vi "Hopping step(linear-XZ).vi"() -> ()   [LabVIEW 2014]
uses:
  <vilib>/Platform/TimedLoop/XDataNode/timing_clust.ctl
  <vilib>/Platform/TimedLoop/XDataNode/nitl_modes.ctl
  <vilib>/Platform/TimedLoop/XDataNode/wakeup.ctl
  <vilib>/rvi/Emulation/niFpgaGetClockAttributes.vi
  <vilib>/rvi/Emulation/niFpgaSctlEmulationGetInTimedLoop.vi
  <vilib>/rvi/Emulation/niFpgaEmulationReportErrorSimple.vi
  <vilib>/rvi/eio/common/nirviEmuTemplateMethod_errors.vi
  <vilib>/rvi/Emulation/niFpgaCriticalErrorInLSC.vi
  <vilib>/rvi/interface/RandomDataEmulation/niFpgaRandomDataHandleErrors.vi
  <vilib>/rvi/Emulation/niFpgaProcessEmulError.vi
  <vilib>/eio/EIONode/EIONode.xnode
  <vilib>/Platform/TimedLoop/XDataNode/XDataNode.xnode
  <vilib>/rvi/DataTransferAndStorage/Container/XNode/niFpgaContainer.xnode
  <vilib>/rvi/interface/RandomDataEmulation/nirviRandomDataFpgaReadWriteTemplate.vi
  <vilib>/Platform/TimedLoop/XDataNode/XDNodeRunTimeDep.lvlib
panel:
  out "Waveform Chart":i32(graph)
  out "ZRealPos":i16
  in  "stop":bool
  out "Z":i32(graph)
  in  "ZOffset":i16
  in  "XNum":i16
  in  "XOffset":i16
  in  "XStepIndex":i16
  in  "WhetherDoubleRow?":bool=TRUE
  in  "RelativeWithdraw":i16
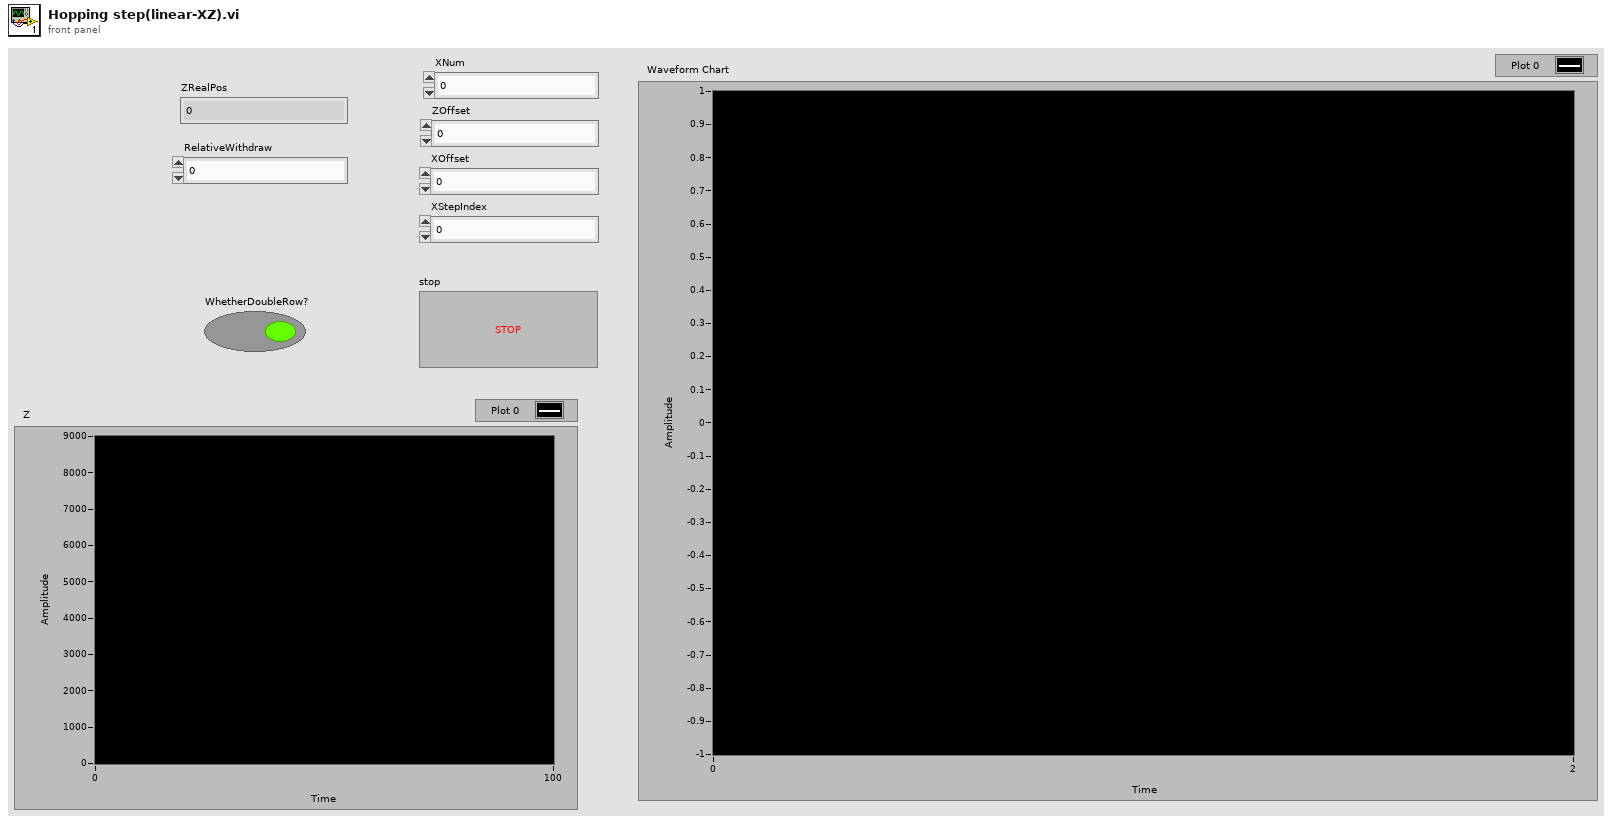
[diagram p1: front panel]
types:
  T1 = typedef "XDNodeRunTimeDep.lvlib/timing_clust.ctl" = cluster{"Expected End [f-1]":u64, "Actual End [f-1]":u64, "Finished Late? [f-1]":bool, "Expected End [i-1]":u64, "Actual End [i-1]":u64, "Finished Late? [i-1]":bool, "Expected Start [i]":u64, "Actual Start [i]":u64, "Expected Start [f]":u64, "Actual Start [f]":u64, "Source Name":string, "Structure Name":string, "Period":i64, "Deadline":i64, "Offset":i64, "Start":i64, "Priority":i32, "Timeout":i32, "Mode":T2, "Wakeup Reason":T3, "Error":errorcluster, "Source Type":string, "Secondary Source Type":string, "Global End Time":u64, "Global Start Time":u64, "Frame Duration":u64, "Iteration Duration":u64, "Assigned CPU":i32, "I/O Scan Engine Mode":u32}
  T2 = typedef "XDNodeRunTimeDep.lvlib/nitl_modes.ctl" = enum32{"No Change", "Process missed periods, maintain original phase", "Discard missed periods, maintain original phase", "Process missed periods, ignore original phase", "Discard missed periods, ignore original phase"}
  T3 = typedef "XDNodeRunTimeDep.lvlib/wakeup.ctl" = enum32{"Normal", "Aborted", "Asynchronous wakeup", "Timing source error", "Timed loop error", "Timeout"}
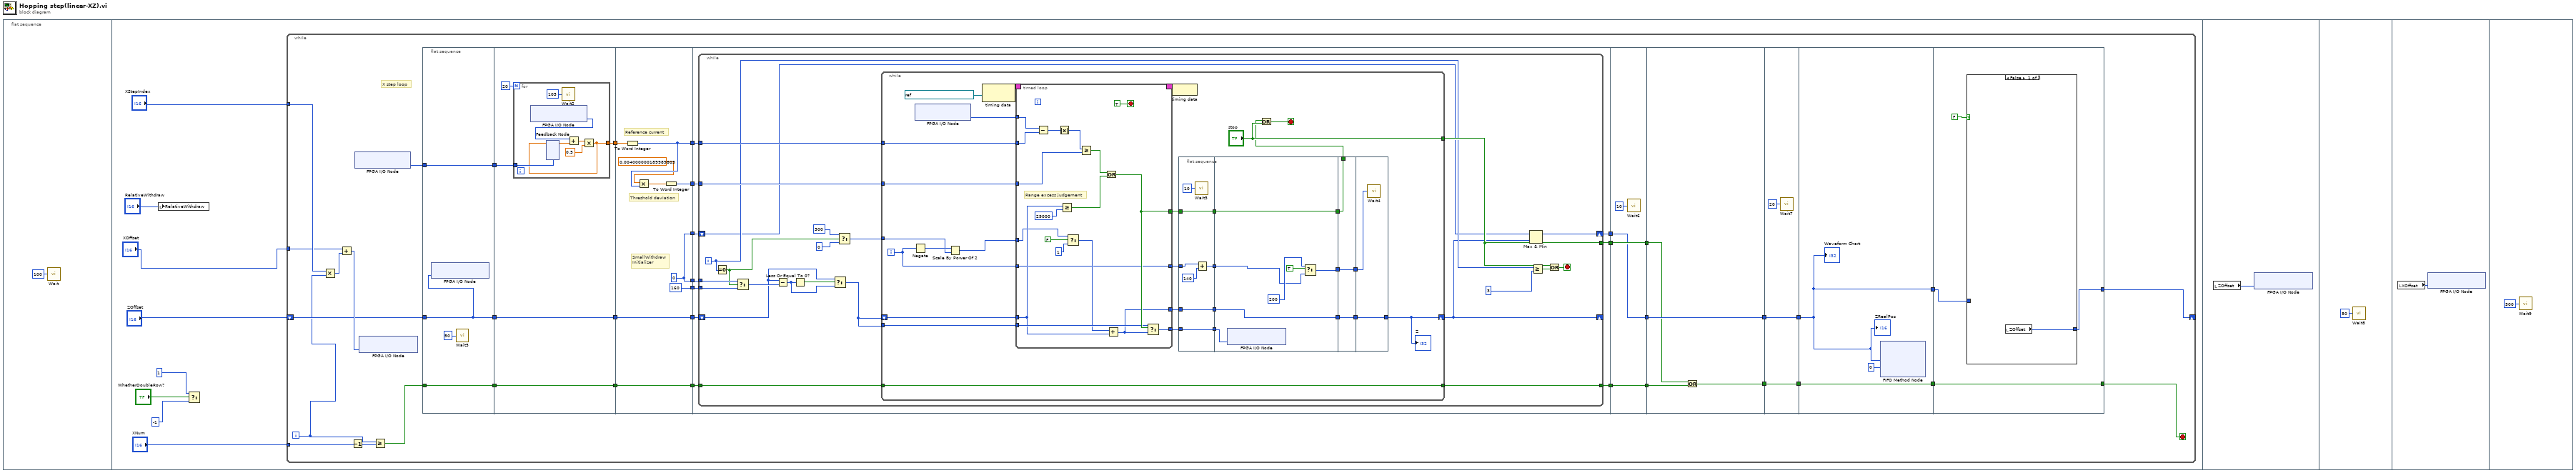
[diagram p0: block diagram]
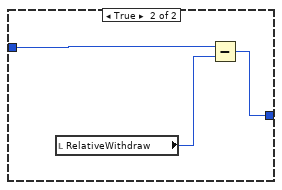
[diagram p2: hidden frame]
diagram:
  n1 = flat-sequence {
    frame #0 {
      n2 = call "Wait"("Count(mSec)"=u32 100 ("Count(uSec)")) -> ()  [unwired: 1 out]
    }
    frame #1 {
      n3 = local write "RelativeWithdraw"("RelativeWithdraw") -> ()
      n4 = Select(t=i16 1, s="WhetherDoubleRow?", f=i16 -1) -> ()  [unwired: 1 out]
      n5 = while {
        tunnel: "XNum" -> [w22]
        tunnel: "XStepIndex" -> [w23]
        shift-right: [w10] -> _
        shift-left: "ZOffset" -> [w24]
        tunnel: "XOffset" -> [w13]
        i -> [w14]
        stop <- w33 stop-if-true
        # "X step loop"
        n6 = Multiply(x=w23, y=w14) -> (x*y=w28:i32)
        n7 = Add(x=w13, y=w28) -> (x+y=w29:i32)
        n8 = Decrement(x=w22) -> (x-1=w21:i16)
        n9 = xnode "FPGA I/O Node"() -> ("Connector0/AI1"=w40:i16)  [unwired: 1 in, 1 out]
        n10 = xnode "FPGA I/O Node"("Connector0/AO2"=w29) -> ()  [unwired: 1 in, 1 out]
        n11 = Greater Or Equal?(x=w14, y=w21) -> (x >= y?=w20:bool)
        n12 = flat-sequence {
          tunnel: [w49] -> w45
          tunnel: w40 -> [w49]
          tunnel: [w48] -> w30
          tunnel: w24 -> [w48]
          tunnel: w20 -> [w47]
          tunnel: [w47] -> w19
          tunnel: w45 -> [w55]
          tunnel: [w53] -> w44
          tunnel: [w52] -> w31
          tunnel: w30 -> [w52]
          tunnel: w19 -> [w51]
          tunnel: [w51] -> w18
          tunnel: [w65] -> w46
          tunnel: w44 -> [w71]
          tunnel: [w70] -> w43
          tunnel: [w67] -> w42
          tunnel: [i16 160] -> w32
          tunnel: w31 -> [w65]
          tunnel: [w64] -> w27
          tunnel: [w64] -> w26
          tunnel: w18 -> [w63]
          tunnel: [w63] -> w17
          tunnel: w42 -> [w79]
          tunnel: w43 -> [w80]
          tunnel: w46 -> [w81]
          tunnel: [w78] -> w36
          tunnel: w32 -> [w77]
          tunnel: w27 -> [w76]
          tunnel: w26 -> [w75]
          tunnel: [w74] -> w25
          tunnel: w17 -> [w73]
          tunnel: [w72] -> w15
          tunnel: [w180] -> w41
          tunnel: [w181] -> w37
          tunnel: w36 -> [w181]
          tunnel: w25 -> [w180]
          tunnel: [w179] -> w16
          tunnel: w15 -> [w179]
          tunnel: w41 -> [w186]
          tunnel: [w186] -> w39
          tunnel: w37 -> [w185]
          tunnel: [w184] -> w34
          tunnel: w16 -> [w183]
          tunnel: w39 -> [w188]
          tunnel: [w188] -> w38
          tunnel: [w187] -> w35
          tunnel: w34 -> [w187]
          tunnel: w38 -> [w190]
          tunnel: w35 -> [w191]
          tunnel: [w191] -> w12
          tunnel: [w190] -> w11
          tunnel: [w194] -> w10
          tunnel: [w196] -> w33
          tunnel: w12 -> [w196]
          tunnel: w11 -> [w193]
          frame #0 {
            n13 = xnode "FPGA I/O Node"("Connector0/AO0"=w48) -> ()  [unwired: 1 in, 1 out]
            n14 = call "Wait5"("Count(uSec)"=u32 50) -> ()  [unwired: 1 out]
          }
          frame #1 {
            n15 = for {
              N: 20 -> [_]
              tunnel: w55 -> [w61]
              tunnel: [w56] -> w53
              n16 = xnode "FPGA I/O Node"() -> ("Connector0/AI1"=w59:i16)  [unwired: 1 in, 1 out]
              n17 = feedback #1(w61) -> (w60:sgl)
              n18 = call "Wait2"("Count(uSec)"=u32 105) -> ()  [unwired: 1 out]
              n19 = Add(x=w59, y=w60) -> (x+y=w58:sgl)
              n20 = Multiply(x=w58, y=sgl 0.5) -> (x*y=w56:sgl)
              n21 = feedback-in #1(w56) -> ()
            }
          }
          frame #2 {
            w64 = i16 0
            # "SmallWithdraw\nInitializer"
            # "Threshold deviation"
            # "Reference current"
            n22 = To Word Integer(number=w71) -> (16bit integer=w70:i16)
            n23 = Multiply(x=sgl 0.004, y=w70) -> (x*y=w68:sgl)
            n24 = To Word Integer(number=w68) -> (16bit integer=w67:i16)
          }
          frame #3 {
            n25 = while {
              tunnel: w80 -> [w104]
              tunnel: w79 -> [w103]
              tunnel: [w100] -> w78
              tunnel: w77 -> [w98]
              shift-right: [w90] -> _
              shift-left: w81 -> [w95]
              tunnel: w76 -> [w92]
              shift-right: [w89] -> w74
              shift-left: w75 -> [w91]
              tunnel: w73 -> [w85]
              tunnel: [w84] -> w72
              i -> [w99]
              stop <- w102 stop-if-true
              n26 = Equal To 0?(x=w99) -> (x = 0?=w82:bool)
              n27 = Select(t=w92, s=w82, f=w98) -> (s? t:f=w97:i16)
              n28 = Subtract(x=w95, y=w97) -> (x-y=w94:i32)
              n29 = Less Or Equal To 0?(x=w94) -> (x <= 0?=w96:bool)
              n30 = Select(t=w95, s=w96, f=w94) -> (s? t:f=w93:i32)
              n31 = Select(t=i16 300, s=w82, f=i16 0) -> (s? t:f=w86:i16)
              n32 = while {
                tunnel: w104 -> [w127]
                tunnel: w103 -> [w129]
                tunnel: ["stop"] -> w100
                shift-right: [w118] -> w90
                shift-left: w93 -> [w124]
                tunnel: w93 -> [w121]
                tunnel: w86 -> [w108]
                tunnel: w85 -> [w105]
                tunnel: [w105] -> w84
                i -> [w106]
                stop <- w131 stop-if-true
                n33 = Negate(x=w106) -> (-x=w109:i32)
                n34 = xnode "FPGA I/O Node"() -> ("Connector0/AI1"=w128:i16)  [unwired: 1 in, 1 out]
                n35 = Scale By Power Of 2(n=w109, x=w108) -> (x*2^n=w107:i16)
                n36 = node-c288(refnum<k21> "40 MHz Onboard Clock" ("Source Name")) -> (w134:T1)
                n37 = timed-loop {
                  timing: w134 -> [_]
                  timing-out: [_] -> w133
                  tunnel: w127 -> [w170]
                  tunnel: w129 -> [w156]
                  tunnel: w128 -> [w171]
                  tunnel: [w166] -> w125
                  tunnel: [w165] -> w123
                  tunnel: w124 -> [w162]
                  tunnel: w121 -> [w164]
                  tunnel: [w161] -> w120
                  tunnel: w107 -> [w157]
                  tunnel: [w158] -> w110
                  tunnel: w106 -> [w158]
                  stop <- TRUE stop-if-true
                  # "Range excess judgement"
                  n38 = Subtract(x=w171, y=w170) -> (x-y=w155:i16)
                  n39 = Absolute Value(x=w155) -> (abs(x)=w169:i16)
                  n40 = Greater Or Equal?(x=w162, y=i16 29000) -> (x >= y?=w167:bool)
                  n41 = Select(t=w157, s=FALSE, f=1) -> (s? t:f=w159:i32)
                  n42 = Greater Or Equal?(x=w169, y=w156) -> (x >= y?=w168:bool)
                  n43 = Or(x=w168, y=w167) -> (x .or. y?=w165:bool)
                  n44 = Add(x=w159, y=w162) -> (x+y=w161:i32)
                  n45 = Select(t=w164, s=w165, f=w161) -> (s? t:f=w166:i32)
                }
                n46 = node-c288(w133) -> ()
                n47 = flat-sequence {
                  tunnel: [w140] -> w126
                  tunnel: w125 -> [w140]
                  tunnel: w123 -> [w139]
                  tunnel: [w139] -> w122
                  tunnel: w120 -> [w138]
                  tunnel: [w138] -> w119
                  tunnel: [w136] -> w111
                  tunnel: w110 -> [w137]
                  tunnel: w126 -> [w146]
                  tunnel: [w148] -> w117
                  tunnel: w122 -> [w147]
                  tunnel: w119 -> [w148]
                  tunnel: [w147] -> w115
                  tunnel: [w144] -> w112
                  tunnel: w111 -> [w143]
                  tunnel: w117 -> [w151]
                  tunnel: [w151] -> w116
                  tunnel: w115 -> [w150]
                  tunnel: [w150] -> w114
                  tunnel: [w149] -> w113
                  tunnel: w112 -> [w149]
                  tunnel: w116 -> [w153]
                  tunnel: [w153] -> w118
                  tunnel: w113 -> [w152]
                  frame #0 {
                    n48 = call "Wait3"("Count(uSec)"=u32 10) -> ()  [unwired: 1 out]
                    n49 = Add(x=w137, y=140) -> (x+y=w136:i32)
                  }
                  frame #1 {
                    n50 = xnode "FPGA I/O Node"("Connector0/AO0"=w146) -> ()  [unwired: 1 in, 1 out]
                    n51 = Select(t=i16 200, s=TRUE, f=w143) -> (s? t:f=w144:i32)
                  }
                  frame #2 {
                  }
                  frame #3 {
                    n52 = call "Wait4"("Count(uSec)"=w152) -> ()  [unwired: 1 out]
                  }
                }
                n53 = Or(x=w114, y="stop") -> (x .or. y?=w131:bool)
                "Z" <- w118
              }
              n54 = Max & Min(x=w91, y=w90) -> (max(x,y)=w89:i32)  [unwired: 1 out]
              n55 = Greater Or Equal?(x=w99, y=3) -> (x >= y?=w101:bool)
              n56 = Or(x=w100, y=w101) -> (x .or. y?=w102:bool)
            }
          }
          frame #4 {
            n57 = call "Wait6"("Count(uSec)"=u32 10) -> ()  [unwired: 1 out]
          }
          frame #5 {
            n58 = Or(x=w185, y=w183) -> (x .or. y?=w184:bool)
          }
          frame #6 {
            n59 = call "Wait7"("Count(uSec)"=u32 20) -> ()  [unwired: 1 out]
          }
          frame #7 {
            n60 = xnode ("FIFO Method Node")("Element"=w190, "Timeout"=0) -> ()  [unwired: 1 in, 2 out]
            "Waveform Chart" <- w190
            "ZRealPos" <- w190
          }
          frame #8 {
            n61 = case shown="False" FALSE {
              tunnel: w193 -> [_ w200]
              tunnel: [w197 w198] -> w194
              frame False {
                n62 = local read "ZOffset"() -> (w197:i16)
              }
              frame True {
                n63 = local read "RelativeWithdraw"() -> (w199:i16)
                n64 = Subtract(x=w200, y=w199) -> (x-y=w198:i32)
              }
            }
          }
        }
      }
    }
    frame #2 {
      n65 = local read "ZOffset"() -> (w201:i16)
      n66 = xnode "FPGA I/O Node"("Connector0/AO0"=w201) -> ()  [unwired: 1 in, 1 out]
    }
    frame #3 {
      n67 = call "Wait8"("Count(uSec)"=u32 50) -> ()  [unwired: 1 out]
    }
    frame #4 {
      n68 = local read "XOffset"() -> (w203:i16)
      n69 = xnode "FPGA I/O Node"("Connector0/AO2"=w203) -> ()  [unwired: 1 in, 1 out]
    }
    frame #5 {
      n70 = call "Wait9"("Count(uSec)"=u32 500) -> ()  [unwired: 1 out]
    }
  }
